vi "Curtin1_ViewMics.vi"(11 "Settings":T1={"Name of test"="ScratchPad", "Date"=timestamp(3622387832 s since 1904-01-01), "Location"="Home", "Template"="ScratchPad", "Soundcard"="Babyface Pro (71982712)", "resolution"=32, "Sampling rate"=48000, "Ch1 Gain "=15.0, "Ch2 Gain"=20.0, "Sample time (s)"=0.3, "Pre-trigger (s)"=0.001, "Hammer Threshold"=0.05, "Positions"=1, "Taps/Position"=5, "Set Names"="H", "Freq resolution"=1.0, "Hammer cutoff"=0.03, "Mic cutoff"=0.1, "Double bounce "=0.01, "Hammer Cal"=1.0, "dB Offset"=0.0, "Accel Cal"=1.0, "Vibrometer Cal"=20.0, "Mic Cal"=49.38, "Output"=2, "Voltage Cal"=13.4, "Vibrometer Port"="ASRL27::INSTR", "Range"=4, "High Pass"=2, "Bandwidth"=4, "X Range"=[{"Minimum"=200.0, "Maximum"=10000.0, "Increment"=10.0, "Minor Increment"=100.0, "Start"=200.0}, {"Minimum"=0.0, "Maximum"=0.05, "Increment"=0.025, "Minor Increment"=0.0025, "Start"=0.0}, {"Minimum"=0.0, "Maximum"=0.3, "Increment"=0.1, "Minor Increment"=0.01, "Start"=0.0}, {"Minimum"=200.0, "Maximum"=10000.0, "Increment"=10.0, "Minor Increment"=100.0, "Start"=1000.0}], "Y Range"=[{"Minimum"=-25.0, "Maximum"=0.0, "Increment"=5.0, "Minor Increment"=1.0, "Start"=-25.0}, {"Minimum"=-0.01, "Maximum"=0.1, "Increment"=0.02, "Minor Increment"=0.005, "Start"=0.0}, {"Minimum"=-0.1, "Maximum"=0.1, "Increment"=0.05, "Minor Increment"=0.01, "Start"=-0.1}, {"Minimum"=-61.0, "Maximum"=-21.0, "Increment"=2.0, "Minor Increment"=0.5, "Start"=-60.0}], "dB Spread"=40.0, "Trigger"=0, "Ch_1"=2, "Ch_2"=1, "flip?"=FALSE, "60Hz"=FALSE, "Time offset"=0.0, "Piezo Cal"=1.0, "Default Notes"="", "Tom"=FALSE} {"Ch_2" min=1 step=1; "Ch_1" min=1 max=100 step=1; "Trigger" items=["Hammer (force)", "Self-tap", "Spacebar"]; "Bandwidth" items=["1 kHz"=1, "5 kHz"=5, "10 kHz"=10, "25 kHz"=25, "50 kHz"=50, "100 kHz"=100]; "High Pass" items=["Off", "13 Hz", "104 Hz"]; "Range" items=["10 mm/s"=1, "20 mm/s"=2, "50 mm/s"=5, "100 mm/s"=10, "200 mm/s"=20, "500 mm/s"=50, "1 m/s"=100, "2 m/s"=200]; "Output" items=["Accelerometer", "Speed (from acceleration)", "Microphone", "Vibrometer", "Piezo"]; "Voltage Cal" format="%#_13g"; "Ch2 Gain" format="%#_13g"; "Ch1 Gain" format="%#_13g"; "Double bounce" min=0.0; "Mic cutoff" min=0.0 format="%#_4g"; "Hammer cutoff" min=0.0 format="%#_4g"; "Freq resolution" min=0.0; "Pre-trigger (s)" format="%#_13g"; "Date" format="%<%H:%M\n%d/%m/%y>T"; "resolution" items=["16 bit"=16, "24 bit"=24, "32 bit"=32]; "Sampling rate" items=["22050 samp/s"=22050, "44100 samp/s"=44100, "48000 samp/s"=48000]}) -> (3 "Settings Out":T1={"Name of test"="ScratchPad", "Date"=timestamp(3622387832 s since 1904-01-01), "Location"="Home", "Template"="ScratchPad", "Soundcard"="Babyface Pro (71982712)", "resolution"=32, "Sampling rate"=48000, "Ch1 Gain "=15.0, "Ch2 Gain"=20.0, "Sample time (s)"=0.3, "Pre-trigger (s)"=0.001, "Hammer Threshold"=0.05, "Positions"=1, "Taps/Position"=5, "Set Names"="H", "Freq resolution"=1.0, "Hammer cutoff"=0.03, "Mic cutoff"=0.1, "Double bounce "=0.01, "Hammer Cal"=1.0, "dB Offset"=0.0, "Accel Cal"=1.0, "Vibrometer Cal"=20.0, "Mic Cal"=49.38, "Output"=2, "Voltage Cal"=13.4, "Vibrometer Port"="ASRL27::INSTR", "Range"=4, "High Pass"=2, "Bandwidth"=4, "X Range"=[{"Minimum"=200.0, "Maximum"=10000.0, "Increment"=10.0, "Minor Increment"=100.0, "Start"=200.0}, {"Minimum"=0.0, "Maximum"=0.05, "Increment"=0.025, "Minor Increment"=0.0025, "Start"=0.0}, {"Minimum"=0.0, "Maximum"=0.3, "Increment"=0.1, "Minor Increment"=0.01, "Start"=0.0}, {"Minimum"=200.0, "Maximum"=10000.0, "Increment"=10.0, "Minor Increment"=100.0, "Start"=1000.0}], "Y Range"=[{"Minimum"=-25.0, "Maximum"=0.0, "Increment"=5.0, "Minor Increment"=1.0, "Start"=-25.0}, {"Minimum"=-0.01, "Maximum"=0.1, "Increment"=0.02, "Minor Increment"=0.005, "Start"=0.0}, {"Minimum"=-0.1, "Maximum"=0.1, "Increment"=0.05, "Minor Increment"=0.01, "Start"=-0.1}, {"Minimum"=-61.0, "Maximum"=-21.0, "Increment"=2.0, "Minor Increment"=0.5, "Start"=-60.0}], "dB Spread"=40.0, "Trigger"=0, "Ch_1"=2, "Ch_2"=1, "flip?"=FALSE, "60Hz"=FALSE, "Time offset"=0.0, "Piezo Cal"=1.0, "Default Notes"="", "Tom"=FALSE} {"Ch_2" min=1 step=1; "Ch_1" min=1 max=100 step=1; "Trigger" items=["Hammer (force)", "Self-tap", "Spacebar"]; "Bandwidth" items=["1 kHz"=1, "5 kHz"=5, "10 kHz"=10, "25 kHz"=25, "50 kHz"=50, "100 kHz"=100]; "High Pass" items=["Off", "13 Hz", "104 Hz"]; "Range" items=["10 mm/s"=1, "20 mm/s"=2, "50 mm/s"=5, "100 mm/s"=10, "200 mm/s"=20, "500 mm/s"=50, "1 m/s"=100, "2 m/s"=200]; "Output" items=["Accelerometer", "Speed (from acceleration)", "Microphone", "Vibrometer", "Piezo"]; "Voltage Cal" format="%#_13g"; "Ch2 Gain" format="%#_13g"; "Ch1 Gain" format="%#_13g"; "Double bounce" min=0.0; "Mic cutoff" min=0.0 format="%#_4g"; "Hammer cutoff" min=0.0 format="%#_4g"; "Freq resolution" min=0.0; "Pre-trigger (s)" format="%#_13g"; "Date" format="%<%H:%M\n%d/%m/%y>T"; "resolution" items=["16 bit"=16, "24 bit"=24, "32 bit"=32]; "Sampling rate" items=["22050 samp/s"=22050, "44100 samp/s"=44100, "48000 samp/s"=48000]})   [LabVIEW 2022 SP3]
uses:
  PreferencesControl.ctl
  <extravilib>/ChannelInstances/Lossy Stream-a[.](wfm(dbl))/Read With Abort.vi
  <extravilib>/ChannelInstances/Lossy Stream-a[.](wfm(dbl))/EndpointRead.vi
  Mic/Mic_Global.vi
  <extravilib>/ChannelInstances/Lossy Stream-a[.](wfm(dbl))/Instantiate.vi
  <extravilib>/ChannelInstances/Lossy Stream-a[.](wfm(dbl))/)Channel.vi
  <resource>/ChannelSupport/_ChannelSupport/WaitIfNeeded.vi
  <extravilib>/ChannelInstances/Lossy Stream-a[.](wfm(dbl)).lvlib
panel:
  in  "dB Spread":dbl=40.0
  in  "rescale Y 2":bool
  out "Hammer Spectrum":cluster{dbl, "df":dbl, "FFT {X}":dbl[]}[](graph)
  out "Average FRF":cluster{dbl, "df":dbl, dbl[]}[](graph)
  in  "OpenVibrometer":bool
  in  "rescale Y":bool
  in  "View":u16(ring) items=["Raw", "Volts", "Units (Pa, N, etc)"]
  out "Microphone Data":waveform(dbl)[](graph)
  out "Hammer Data":waveform(dbl)[](graph)
  in  "stop":bool
  # "Hz"
  # "dB"
  # "dB"
  # "sec"
  # "sec"
  # "mV/Pa"
  # "mV/m/s2"
  # "mV/mm/s"
  # "V/N"
  # "sec"
  # "sec"
  # "mV/N"
  # "a.u."
  # "a.u."
  # "sec"
  # "Hz"
  # "dB"
  # "dB"
  # "sec"
  # "sec"
  # "mV/Pa"
  # "mV/m/s2"
  # "mV/mm/s"
  # "V/N"
  # "sec"
  # "sec"
  # "mV/N"
  # "a.u."
  # "a.u."
  # "sec"
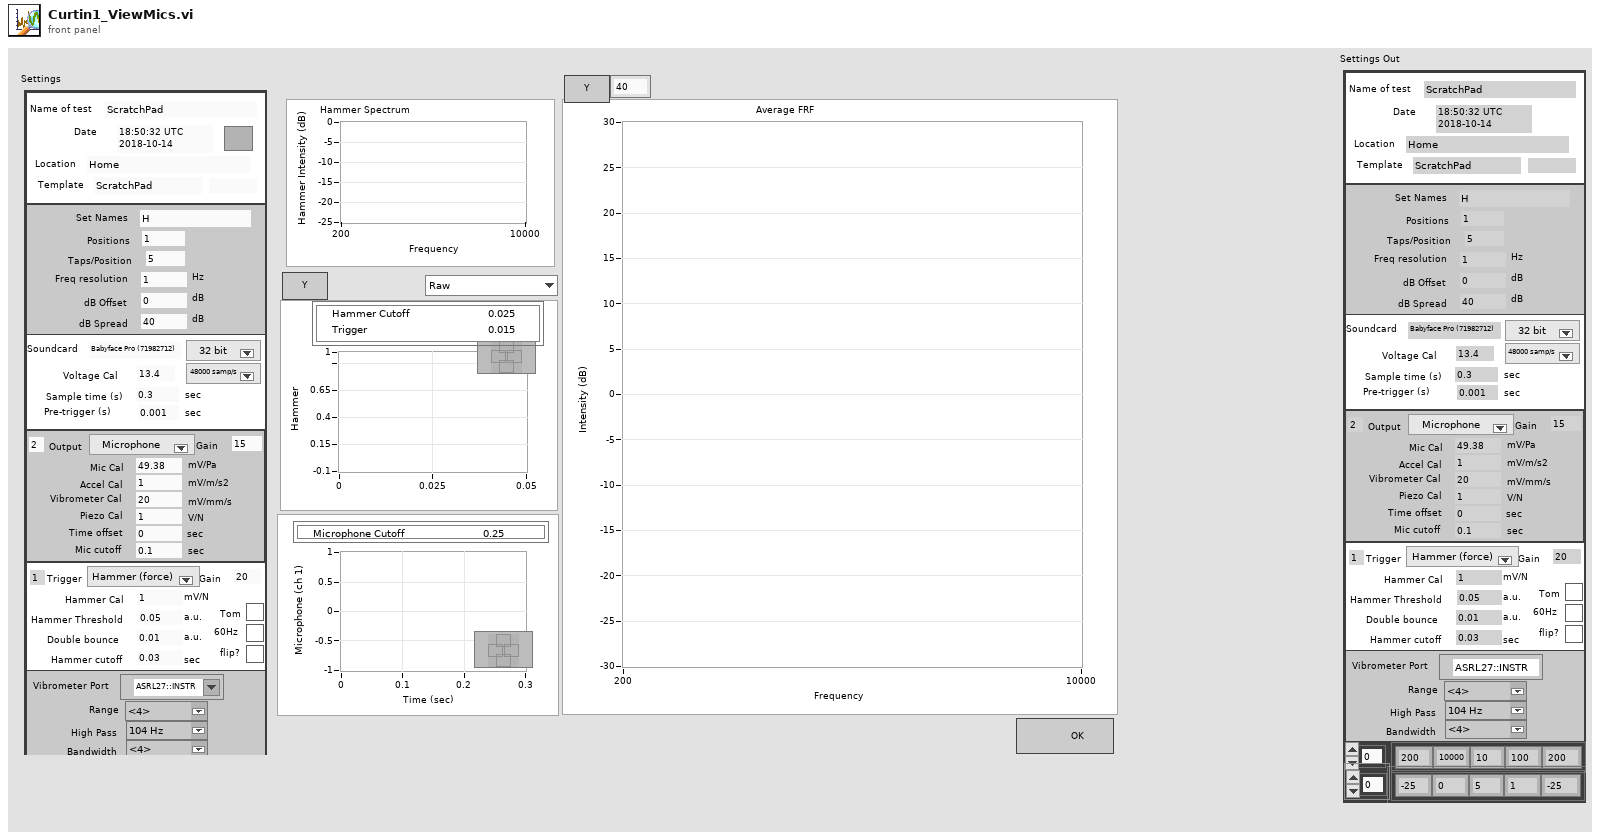
[diagram p1: front panel]
types:
  T1 = typedef "PreferencesControl.ctl" = cluster{"Name of test":string, "Date":timestamp, "Location":string, "Template":string, "Soundcard":string, "resolution":u16, "Sampling rate":u16, "Ch1 Gain ":dbl, "Ch2 Gain":dbl, "Sample time (s)":dbl, "Pre-trigger (s)":dbl, "Hammer Threshold":dbl, "Positions":i16, "Taps/Position":i16, "Set Names":string, "Freq resolution":dbl, "Hammer cutoff":dbl, "Mic cutoff":dbl, "Double bounce ":dbl, "Hammer Cal":dbl, "dB Offset":dbl, "Accel Cal":dbl, "Vibrometer Cal":dbl, "Mic Cal":dbl, "Output":u16, "Voltage Cal":dbl, "Vibrometer Port":refnum<visa-resource-name>, "Range":u16, "High Pass":u16, "Bandwidth":u16, "X Range":cluster{"Minimum":dbl, "Maximum":dbl, "Increment":dbl, "Minor Increment":dbl, "Start":dbl}[], "Y Range":cluster{"Minimum":dbl, "Maximum":dbl, "Increment":dbl, "Minor Increment":dbl, "Start":dbl}[], "dB Spread":dbl, "Trigger":u16, "Ch_1":u8, "Ch_2":u8, "flip?":bool, "60Hz":bool, "Time offset":dbl, "Piezo Cal":dbl, "Default Notes":string, "Tom":bool}
  T2 = enum16{"Initialize", "Free run", "One Shot - waiting", "One Shot - triggered", "Wait", "Close"}
  T3 = cluster{"Minimum":dbl, "Maximum":dbl, "Increment":dbl, "Minor Increment":dbl, "Start":dbl}[]
  T4 = typedef "Sound Input Task ID.ctl" = u32
  T5 = cluster{"task ID":T4, "Num Pts":i32, "timeout":dbl, "FIFO":i32, "Double Bounce":dbl}
  T6 = typedef "Lossy Stream-a[.](wfm(dbl)).lvlib/)Channel.ctl" = refnum<queue>
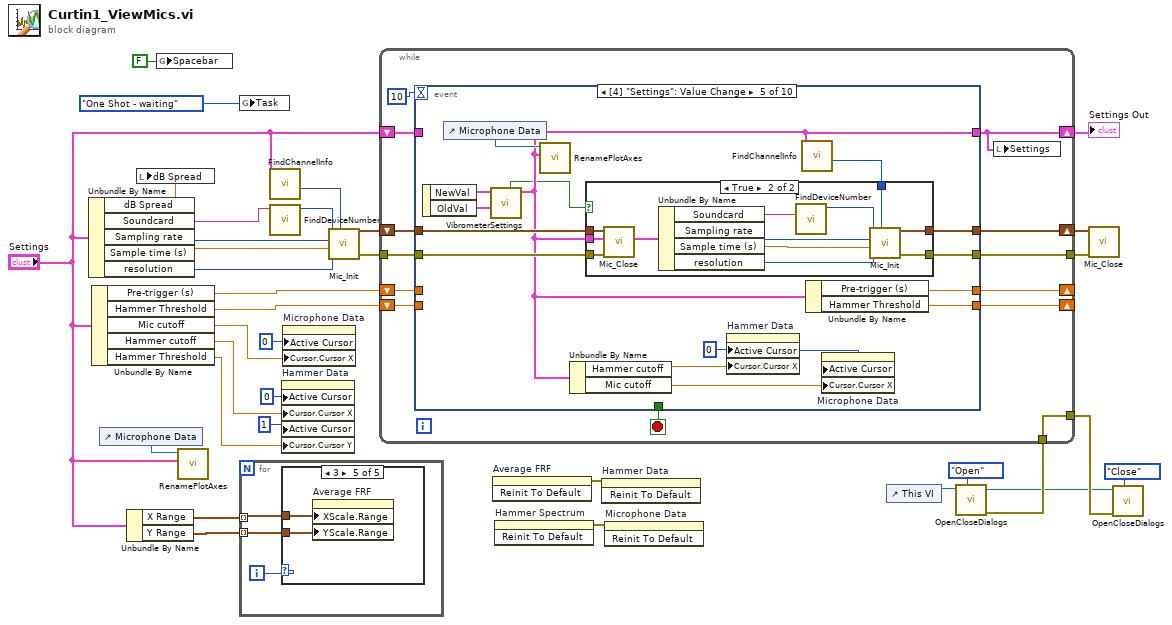
[diagram p0: block diagram]
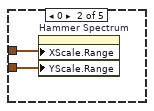
[diagram p3: hidden frame]
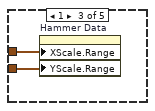
[diagram p4: hidden frame]
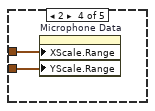
[diagram p5: hidden frame]
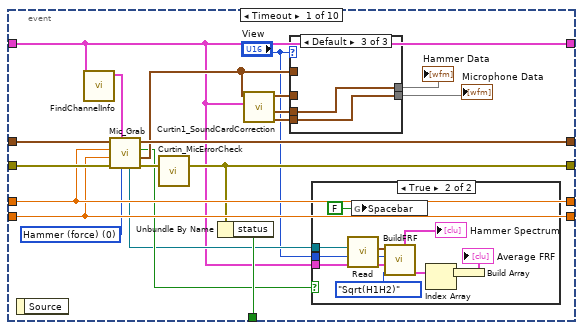
[diagram p6: hidden frame]
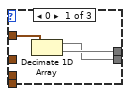
[diagram p8: hidden frame]
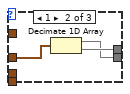
[diagram p9: hidden frame]
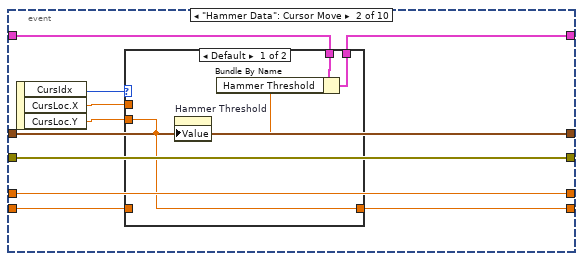
[diagram p10: hidden frame]
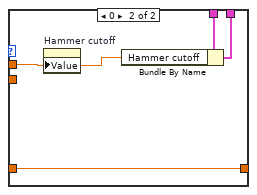
[diagram p11: hidden frame]
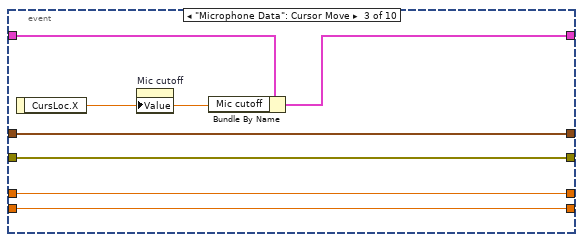
[diagram p12: hidden frame]
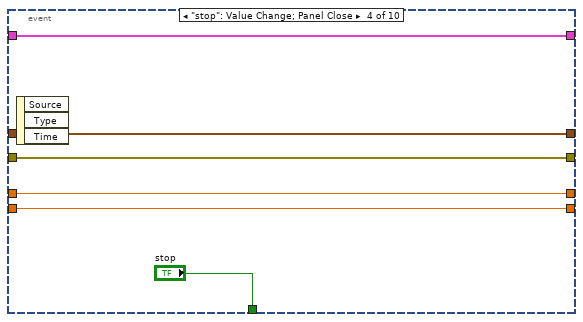
[diagram p13: hidden frame]
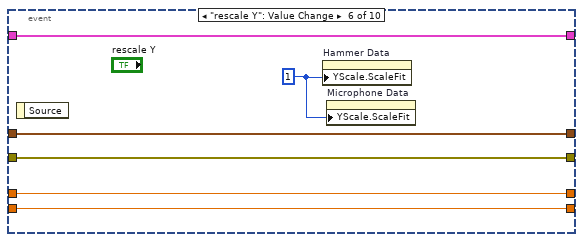
[diagram p15: hidden frame]
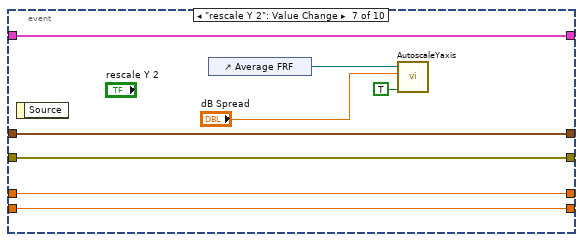
[diagram p16: hidden frame]
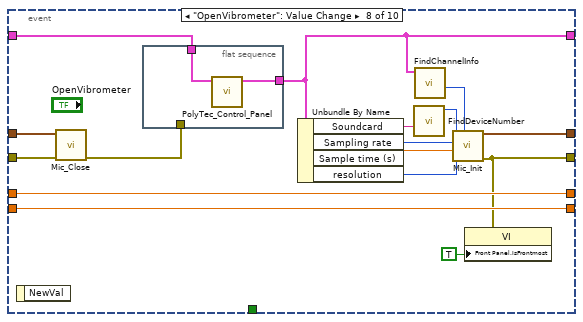
[diagram p17: hidden frame]
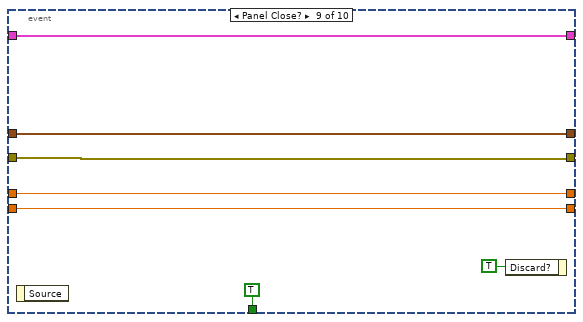
[diagram p18: hidden frame]
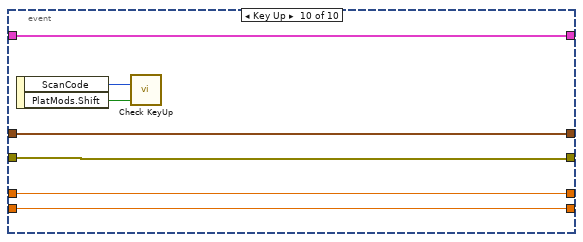
[diagram p19: hidden frame]
diagram:
  n1 = Unbundle By Name("Settings") -> ("dB Spread"=w8:dbl, "Soundcard"=w30:string, "Sampling rate"=w28:u16, "Sample time (s)"=w27:dbl, "resolution"=w26:u16)
  n2 = Unbundle By Name("Settings") -> ("Pre-trigger (s)"=w34:dbl, "Hammer Threshold"=w33:dbl, "Mic cutoff"=w18:dbl, "Hammer cutoff"=w21:dbl, "Hammer Threshold"=w12:dbl)
  n3 = control-ref of="Microphone Data"() -> (w17:refnum<vi>)
  n4 = Unbundle By Name("Settings") -> ("X Range"=w16:T3, "Y Range"=w15:T3)
  n5 = local write "dB Spread"(w8) -> ()
  n6 = global write "Mic_Global.vi" "Spacebar"(FALSE ("Spacebar")) -> ()
  n7 = call "RenamePlotAxes.vi"("Settings"="Settings", "WaveformGraph in"=w17) -> ()  [unwired: 10 in]
  n8 = global write "Mic_Global.vi" "Task"(T2."One Shot - waiting" ("Task")) -> ()
  n9 = for {
    tunnel: w16 -> [w36] mode=indexing
    tunnel: w15 -> [w35] mode=indexing
    i -> [w37]
    n10 = case shown="3" w37 {
      tunnel: w36 -> [_ w38 w41 w43 w45]
      tunnel: w35 -> [_ w39 w40 w42 w44]
      frame Default {
      }
      frame 0 {
        n11 = property on="Hammer Spectrum" class="WFGraph (strict)"("XScale.Range"=w38, "YScale.Range"=w39) -> ()  [unwired: 2 in, 2 out]
      }
      frame 1 {
        n12 = property on="Hammer Data" class="WFGraph (strict)"("XScale.Range"=w41, "YScale.Range"=w40) -> ()  [unwired: 2 in, 2 out]
      }
      frame 2 {
        n13 = property on="Microphone Data" class="WFGraph (strict)"("XScale.Range"=w43, "YScale.Range"=w42) -> ()  [unwired: 2 in, 2 out]
      }
      frame 3 {
        n14 = property on="Average FRF" class="WFGraph (strict)"("XScale.Range"=w45, "YScale.Range"=w44) -> ()  [unwired: 2 in, 2 out]
      }
    }
  }
  n15 = call "FindChannelInfo.vi"("Settings"="Settings") -> ("# chans"=w9:u8)  [unwired: 9 in, 1 out]
  n16 = call "FindDeviceNumber.vi"("device"=w30) -> ("device"=w29:u16)  [unwired: 10 in]
  n17 = property on="Hammer Data" class="WFGraph (strict)"("Active Cursor"=u32 0, "Cursor.Cursor X"=w21, "Active Cursor"=u32 1, "Cursor.Cursor Y"=w12) -> ()  [unwired: 2 in, 2 out]
  n18 = property on="Microphone Data" class="WFGraph (strict)"("Active Cursor"=u32 0, "Cursor.Cursor X"=w18) -> ()  [unwired: 2 in, 2 out]
  n19 = call "Mic_Init.vi"("# channels"=w9, "resolution"=w26, "Sample time"=w27, "Sampling rate"=w28, "device"=w29) -> ("error out"=w32:errorcluster, "DAQ Prams"=w31:T5)  [unwired: 5 in]
  n20 = invoke on="Average FRF" class="WFGraph (strict)" method="Reinit To Default"() -> (error out=w14:errorcluster)  [unwired: 3 in, 2 out]
  n21 = invoke on="Hammer Spectrum" class="WFGraph (strict)" method="Reinit To Default"() -> (error out=w13:errorcluster)  [unwired: 3 in, 2 out]
  n22 = invoke on="Hammer Data" class="WFGraph (strict)" method="Reinit To Default"(error in=w14) -> ()  [unwired: 2 in, 3 out]
  n23 = invoke on="Microphone Data" class="WFGraph (strict)" method="Reinit To Default"(error in=w13) -> ()  [unwired: 2 in, 3 out]
  n24 = control-ref of="This VI"() -> (w7:refnum<vi>)
  n25 = call "OpenCloseDialogs.vi"("Task"=enum16{"Open", "Close"}."Open", "VI in"=w7) -> ("error out"=w5:errorcluster, "VI out"=w2:refnum<vi>)  [unwired: 8 in]
  n26 = while {
    tunnel: w32 -> [w56]
    shift-right: [w54] -> w25
    shift-left: w31 -> [w55]
    tunnel: [w53] -> w24
    shift-right: [w52] -> _
    shift-left: w34 -> [w58]
    shift-right: [w51] -> _
    shift-left: w33 -> [w57]
    shift-right: [w47] -> w22
    shift-left: "Settings" -> [w48]
    tunnel: w5 -> [w46]
    tunnel: [w46] -> w3
    stop <- w49 stop-if-true
    n27 = event shown="[4] \"Settings\": Value Change" {
      selector: _ -> [_ _ _ _ _ _ _ _ _ _]
      dyn-events: _ -> [_ _ _ _ _ _ _ _ _ _]
      timeout: 10 -> [_ _ _ _ _ _ _ _ _ _]
      tunnel: w58 -> [w74 w101 w118 w124 _ w157 w165 w183 w191 w199]
      tunnel: w57 -> [w73 w102 w119 w125 _ w156 w164 w182 w190 w198]
      tunnel: w56 -> [w77 w99 w116 w122 w140 w158 w166 w180 w187 w195]
      tunnel: w55 -> [w76 w100 w117 w123 w139 w159 w167 w179 w189 w197]
      tunnel: [w75 w100 w117 w123 w136 w159 w167 w173 w189 w197] -> w54
      tunnel: [w66 w99 w116 w122 w135 w158 w166 w170 w187 w195] -> w53
      tunnel: [w74 w101 w118 w124 w138 w157 w165 w183 w191 w199] -> w52
      tunnel: [w73 w103 w119 w125 w137 w156 w164 w182 w190 w198] -> w51
      tunnel: [w65 _ _ "stop" _ _ _ _ TRUE ("stop") _] -> w49
      tunnel: w48 -> [w60 w97 w115 w120 _ w154 w163 w181 w188 w196]
      tunnel: [w60 w96 w113 w120 w129 w154 w163 w169 w188 w196] -> w47
      event Timeout {
        w64 = u16 0 items=["Hammer (force)", "Self-tap"] ("Input")
        n28 = event-data() -> ()  [unwired: 1 in, 1 out]
        n29 = call "FindChannelInfo.vi"("Settings"=w60) -> ("Info"=w59:cluster{"Ch_1":u8, "Ch_2":u8, "flip?":bool})  [unwired: 9 in, 1 out]
        n30 = call "Mic_Grab.vi"("Input"=w64, "Ports"=w59, "error In"=w77, "Threshold"=w73, "Pre-trigger (s)"=w74, "DAQ Prams"=w76) -> ("error out"=w66:errorcluster, "latest data"=w72:waveform(dbl)[], "Full"=w63:bool, "DAQ Prams"=w75:T5, "Tap"=w62:T6)  [unwired: 1 out]
        n31 = call "Curtin_MicErrorCheck.vi"("error in (no error)"=w66) -> ()  [unwired: 11 in]
        n32 = Unbundle By Name(w66) -> ("status"=w65:bool)
        n33 = call "Curtin1_SoundCardCorrection.vi"("Settings"=w60, "Buffer in"=w72) -> ("Microphone"=w67:waveform(dbl)[], "Hammer"=w68:waveform(dbl)[], "Volts Out"=w69:waveform(dbl)[])  [unwired: 4 in, 3 out]
        n34 = case shown="Default" "View" {
          tunnel: w72 -> [w90 _ _]
          tunnel: [w89 w93 w95] -> w71
          tunnel: [w88 w92 w94] -> w70
          tunnel: w69 -> [_ w91 _]
          tunnel: w68 -> [_ _ w95]
          tunnel: w67 -> [_ _ w94]
          frame 0 {
            n35 = Decimate 1D Array(w90) -> (w88:waveform(dbl)[], w89:waveform(dbl)[])
          }
          frame 1 {
            n36 = Decimate 1D Array(w91) -> (w92:waveform(dbl)[], w93:waveform(dbl)[])
          }
          frame Default {
          }
        }
        "Hammer Data" <- w71
        "Microphone Data" <- w70
        n37 = case shown="True" w63 {
          tunnel: w62 -> [_ w87]
          tunnel: w60 -> [_ w83]
          tunnel: "View" -> [_ w82]
          frame False {
          }
          frame True {
            n38 = call <extravilib>:"Read.vi"("channel"=w87) -> ("element"=w86:waveform(dbl)[])  [unwired: 5 in, 5 out]
            n39 = global write "Mic_Global.vi" "Spacebar"(FALSE ("Spacebar")) -> ()
            n40 = call "BuildFRF.vi"("Method"=enum16{"Sqrt(H1H2)", "H1", "H2"}."Sqrt(H1H2)", "Settings"=w83, "View"=w82, "Data In"=w86) -> ("Average FRF"=w85:cluster{dbl, "df":dbl, dbl[]}[], "Hammer Spectra"=→"Hammer Spectrum":cluster{dbl, "df":dbl, "FFT {X}":dbl[]}[])  [unwired: 2 in, 4 out]
            n41 = Index Array(array=w85) -> (element=w80:cluster{dbl, "df":dbl, dbl[]})  [unwired: 1 in]
            n42 = Build Array(w80) -> (→"Average FRF":cluster{dbl, "df":dbl, dbl[]}[])
          }
        }
      }
      event "Hammer Data": Cursor Move {
        n43 = event-data() -> ("CursIdx"=w105:i32, "CursLoc.X"=w104:dbl, "CursLoc.Y"=w98:dbl)  [unwired: 1 in]
        n44 = case shown="Default" w105 {
          tunnel: w104 -> [_ w109]
          tunnel: [w107 w112] -> w103
          tunnel: w102 -> [_ w112]
          tunnel: w98 -> [w107 _]
          tunnel: w97 -> [w108 w111]
          tunnel: [w106 w110] -> w96
          frame Default {
            n45 = property on="Hammer Threshold" class="DigNum (strict)"("Value"=w107) -> ()  [unwired: 2 in, 2 out]
            n46 = Bundle By Name(cluster=w108, "Hammer Threshold"=w107) -> (w106:T1)
          }
          frame 0 {
            n47 = property on="Hammer cutoff" class="DigNum (strict)"("Value"=w109) -> ()  [unwired: 2 in, 2 out]
            n48 = Bundle By Name(cluster=w111, "Hammer cutoff"=w109) -> (w110:T1)
          }
        }
      }
      event "Microphone Data": Cursor Move {
        n49 = event-data() -> ("CursLoc.X"=w114:dbl)  [unwired: 1 in]
        n50 = property on="Mic cutoff" class="DigNum (strict)"("Value"=w114) -> ()  [unwired: 2 in, 2 out]
        n51 = Bundle By Name(cluster=w115, "Mic cutoff"=w114) -> (w113:T1)
      }
      event "stop": Value Change; Panel Close {
        n52 = event-data() -> ()  [unwired: 1 in, 3 out]
      }
      event Value Change {
        w134 = u32 0 ("Active Cursor")
        n53 = event-data() -> ("NewVal"=w131:T1, "OldVal"=w132:T1)  [unwired: 1 in]
        n54 = control-ref of="Microphone Data"() -> (w133:refnum<vi>)
        n55 = call "VibrometerSettings.vi"("OldVal"=w132, "NewVal"=w131) -> ("Settings"=w129:T1, "update mic"=w126:bool)  [unwired: 5 in, 3 out]
        n56 = call "RenamePlotAxes.vi"("Settings"=w129, "WaveformGraph in"=w133) -> ()  [unwired: 10 in]
        n57 = Unbundle By Name(w129) -> ("Hammer cutoff"=w128:dbl, "Mic cutoff"=w127:dbl)
        n58 = property on="Hammer Data" class="WFGraph (strict)"("Active Cursor"=w134, "Cursor.Cursor X"=w128) -> ()  [unwired: 2 in, 2 out]
        n59 = call "FindChannelInfo.vi"("Settings"=w129) -> ("# chans"=w130:u8)  [unwired: 9 in, 1 out]
        n60 = case shown="True" w126 {
          tunnel: w140 -> [w141 w153]
          tunnel: w139 -> [w142 w152]
          tunnel: [w142 w147] -> w136
          tunnel: [w141 w146] -> w135
          tunnel: w130 -> [_ w144]
          tunnel: w129 -> [_ w143]
          frame False {
          }
          frame True {
            n61 = call "Mic_Close.vi"("error in (no error)"=w153, "DAQ Prams"=w152) -> ()  [unwired: 9 in, 1 out]
            n62 = Unbundle By Name(w143) -> ("Soundcard"=w148:string, "Sampling rate"=w150:u16, "Sample time (s)"=w151:dbl, "resolution"=w145:u16)
            n63 = call "FindDeviceNumber.vi"("device"=w148) -> ("device"=w149:u16)  [unwired: 10 in]
            n64 = call "Mic_Init.vi"("# channels"=w144, "resolution"=w145, "Sample time"=w151, "Sampling rate"=w150, "device"=w149) -> ("error out"=w146:errorcluster, "DAQ Prams"=w147:T5)  [unwired: 5 in]
          }
        }
        n65 = Unbundle By Name(w129) -> ("Pre-trigger (s)"=w138:dbl, "Hammer Threshold"=w137:dbl)
        n66 = property on="Microphone Data" class="WFGraph (strict)"("Active Cursor"=w134, "Cursor.Cursor X"=w127) -> ()  [unwired: 2 in, 2 out]
      }
      event "rescale Y": Value Change {
        w155 = u8 1 ("Y Scale.Scale Fit")
        n67 = event-data() -> ()  [unwired: 1 in, 1 out]
        n68 = property on="Hammer Data" class="WFGraph (strict)"("YScale.ScaleFit"=w155) -> ()  [unwired: 2 in, 2 out]
        n69 = property on="Microphone Data" class="WFGraph (strict)"("YScale.ScaleFit"=w155) -> ()  [unwired: 2 in, 2 out]
      }
      event "rescale Y 2": Value Change {
        n70 = event-data() -> ()  [unwired: 1 in, 1 out]
        n71 = control-ref of="Average FRF"() -> (w160:refnum<vi>)
        n72 = call "AutoscaleYaxis.vi"("Has Coherence in plot?"=TRUE, "dB Range"="dB Spread", "WaveformGraph in"=w160) -> ()  [unwired: 9 in]
      }
      event "OpenVibrometer": Value Change {
        n73 = event-data() -> ()  [unwired: 1 in, 1 out]
        n74 = call "Mic_Close.vi"("error in (no error)"=w180, "DAQ Prams"=w179) -> ("error out"=w172:errorcluster)  [unwired: 9 in]
        n75 = flat-sequence {
          tunnel: w181 -> [w185]
          tunnel: [w184] -> w169
          tunnel: w172 -> [_]
          frame #0 {
            n76 = call "PolyTec_Control_Panel.vi"("Settings in"=w185) -> ("Settings Out"=w184:T1)  [unwired: 8 in, 2 out]
          }
        }
        n77 = Unbundle By Name(w169) -> ("Soundcard"=w175:string, "Sampling rate"=w177:u16, "Sample time (s)"=w178:dbl, "resolution"=w174:u16)
        n78 = call "FindDeviceNumber.vi"("device"=w175) -> ("device"=w176:u16)  [unwired: 10 in]
        n79 = call "FindChannelInfo.vi"("Settings"=w169) -> ("# chans"=w168:u8)  [unwired: 9 in, 1 out]
        n80 = call "Mic_Init.vi"("# channels"=w168, "resolution"=w174, "Sample time"=w178, "Sampling rate"=w177, "device"=w176) -> ("error out"=w170:errorcluster, "DAQ Prams"=w173:T5)  [unwired: 5 in]
        n81 = property class="VI"(error in=w170, "Front Panel.IsFrontmost"=TRUE ("Front Panel Window:Is Frontmost")) -> ()  [unwired: 1 in, 2 out]
      }
      event Panel Close? {
        n82 = event-data() -> ()  [unwired: 1 in, 1 out]
        n83 = event-data("Discard?"=TRUE) -> ()  [unwired: 1 in, 1 out]
      }
      event Key Up {
        n84 = event-data() -> ("ScanCode"=w193:i16, "PlatMods.Shift"=w194:bool)  [unwired: 1 in]
        n85 = call "Check KeyUp.vi"("Shift"=w194, "ScanCode"=w193) -> ()  [unwired: 9 in, 1 out]
      }
    }
    n86 = local write "Settings"(w47) -> ()
  }
  "Settings Out" <- w22
  n87 = call "Mic_Close.vi"("error in (no error)"=w24, "DAQ Prams"=w25) -> ()  [unwired: 9 in, 1 out]
  n88 = call "OpenCloseDialogs.vi"("Task"=enum16{"Open", "Close"}."Close", "error in (no error)"=w3, "VI in"=w2) -> ()  [unwired: 7 in, 2 out]
